vi "Create XNet Frame Name.vi"(8 "error in (no error)":errorcluster, 10 "Source Address":u8, 11 "name":string) -> (0 "error out":errorcluster, 3 "String":string)   [LabVIEW 2013, in "J1939.lvlib"]
uses:
  J1939.lvlib
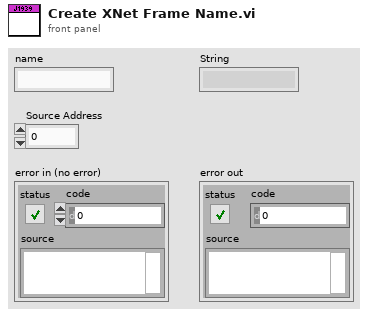
[diagram p1: front panel]
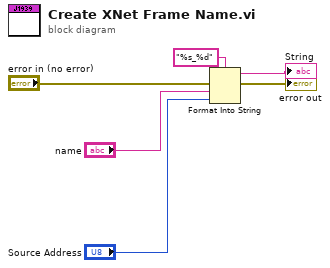
[diagram p0: block diagram]
diagram:
  n1 = Format Into String(format string="%s_%d", error in="error in (no error)", "name", "Source Address") -> (resulting string=→"String":string, error out=→"error out":errorcluster)  [unwired: 1 in]
